vi "Write Status Events.vi"(10 "Status Events":refnum<class "Status Events.lvclass">, 11 "Jenkins Builder in":refnum<class "Jenkins Builder.lvclass">) -> (3 "Jenkins Builder out":refnum<class "Jenkins Builder.lvclass">)   [LabVIEW 2014, in "Jenkins Builder.lvclass"]
uses:
  Jenkins Builder.lvclass
  Shared/Classes/Status Events/Status Events.lvclass
  Jenkins Builder.lvclass/Jenkins Builder.ctl
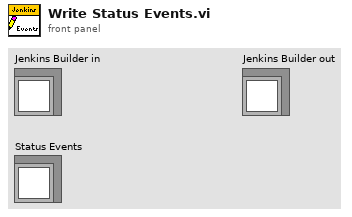
[diagram p1: front panel]
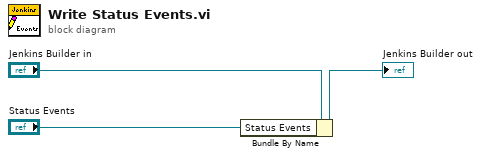
[diagram p0: block diagram]
diagram:
  n1 = Bundle By Name(cluster="Jenkins Builder in", "Status Events"="Status Events") -> (→"Jenkins Builder out":refnum<class "Jenkins Builder.lvclass">)
